vi "Bootstrapping.vi"() -> ()   [LabVIEW 2012]
panel:
  in  "bootstrap script":string="-- This is an example bootstrap script with the optional onfiguration\n-- actions and settings commented out.\n\n-- Substitution of \"\\\" and \"/\" in path strings with the platform path seperator\n-- is enabled by default. Uncomment the line below to disable this behaviour.\n--lv.substitute_separators(false)\n\n-- To globally tune auto-yielding, uncomment the line below and tweak\n-- the timing parameters.\n--lv.setyieldingdefaults(2,0)\n\n-- Specify various configuration settings. When a setting is commented out\n-- or omitted, its current/default value will be used. When the bootstrap\n-- script completes, any changes made to these settings will be reverted.\n-- These settings map to globals \"glb_LuaVIEW Configuration Globals.vi\"\n-- and \"glb_Library Configuration Globals.vi\". See the description of the\n-- variables contained therein for detailed documentation.\nconfigure({\n--[\"bootmode\"]=\"test\"\n--[\"resource base path\"]=lv.app_dir(),\n--[\"time format\"]=\"%Y/%m/%d %H:%M:%S\",\n--[\"persistence path\"]=\"great app\",\n--[\"auto-init registry\"]=true,\n--[\"unload functions ASAP\"]=(app_kind()==\"Run Time System\"),\n--[\"script search directories\"]={\"imports/libraries\",\"imports/configs\"},\n--[\"custom info\"]=\"My great application. (C) GreatWare Inc.\",\n--[\"export timeout\"]=1000,\n--[\"incite timeout\"]=1000,\n--[\"mandatory import script\"]=[[]],\n--[\"task error logger\"]=\"\",\n})\n\n-- Register a selection of public LuaVIEW functions.\nif app_kind()~=\"Run Time System\" then\n    register.public_dir(\"luaview/functions\")\nend\n\n-- Now we can start a script that can assume a proper configuration\n-- and use the public functions that were registered.\n-- Note that a script file can be used instead of an in-line script.\ndo_script(\"startup\",[[\nprint(\"Hello world!\")\nwait(2000)\nprint(\"Goodbye cruel world...\")\n]])\n"
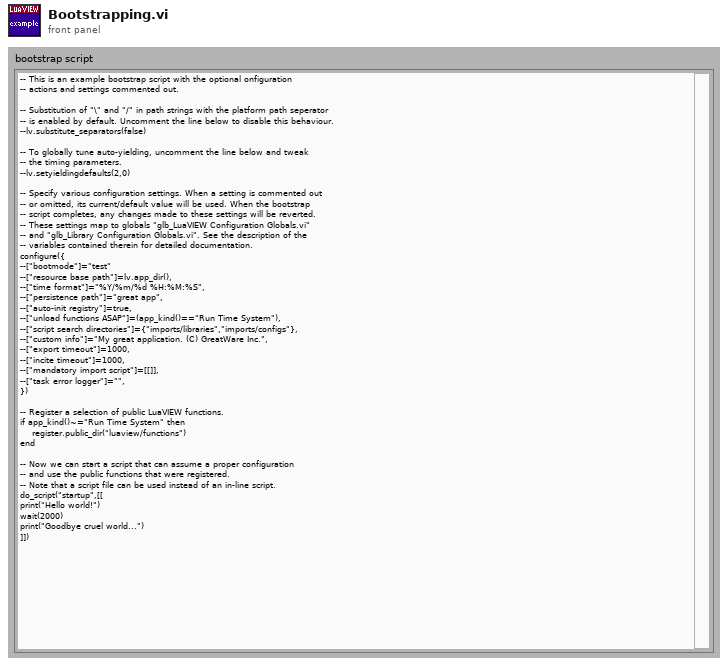
[diagram p1: front panel]
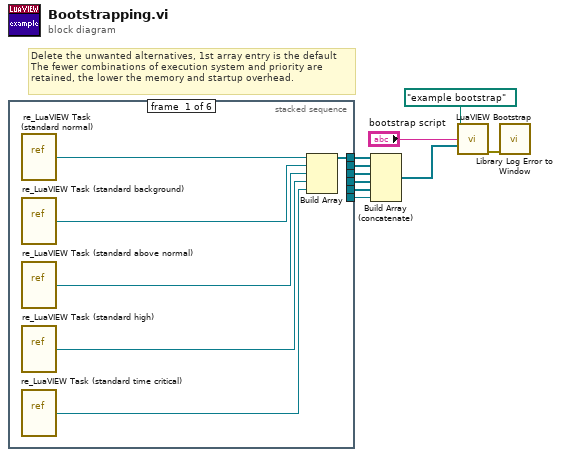
[diagram p0: block diagram]
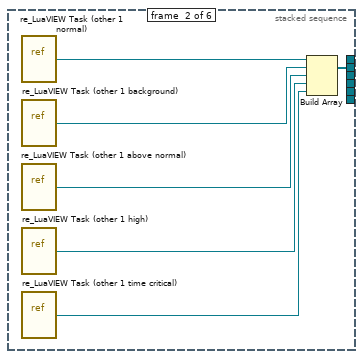
[diagram p2: hidden frame]
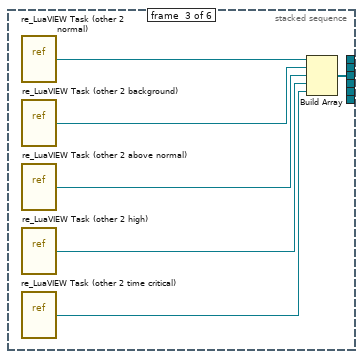
[diagram p3: hidden frame]
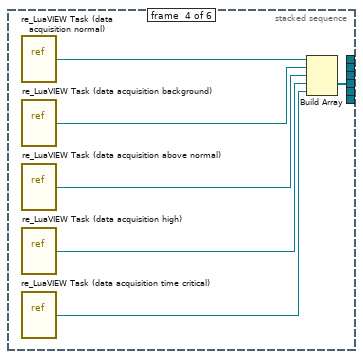
[diagram p4: hidden frame]
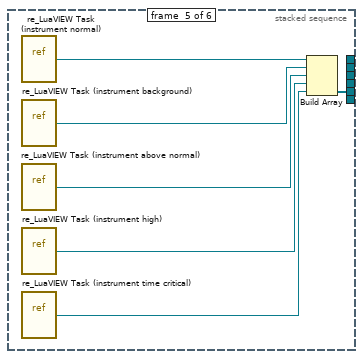
[diagram p5: hidden frame]
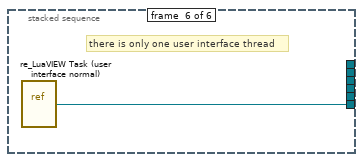
[diagram p6: hidden frame]
diagram:
  # "Delete the unwanted alternatives, 1st array entry is the default\nThe fewer combinations of execution system and priority are\nretained, the lower the memory and startup overhead."
  n1 = stacked-sequence {
    tunnel: [w11 _ _ _ _ _] -> w7
    tunnel: [_ w17 _ _ _ _] -> w6
    tunnel: [_ _ w23 _ _ _] -> w5
    tunnel: [_ _ _ w29 _ _] -> w4
    tunnel: [_ _ _ _ w35 _] -> w3
    tunnel: [_ _ _ _ _ w41] -> w2
    frame #0 {
      n2 = vi-ref "re_LuaVIEW Task (standard normal).vi"() -> ("vi reference"=w16:refnum<vi>)
      n3 = vi-ref "re_LuaVIEW Task (standard background).vi"() -> ("vi reference"=w15:refnum<vi>)
      n4 = vi-ref "re_LuaVIEW Task (standard above normal).vi"() -> ("vi reference"=w14:refnum<vi>)
      n5 = vi-ref "re_LuaVIEW Task (standard high).vi"() -> ("vi reference"=w13:refnum<vi>)
      n6 = vi-ref "re_LuaVIEW Task (standard time critical).vi"() -> ("vi reference"=w12:refnum<vi>)
      n7 = Build Array(w16, w15, w14, w13, w12) -> (w11:refnum<vi>[])
    }
    frame #1 {
      n8 = vi-ref "re_LuaVIEW Task (other 1 normal).vi"() -> ("vi reference"=w22:refnum<vi>)
      n9 = vi-ref "re_LuaVIEW Task (other 1 background).vi"() -> ("vi reference"=w21:refnum<vi>)
      n10 = vi-ref "re_LuaVIEW Task (other 1 above normal).vi"() -> ("vi reference"=w20:refnum<vi>)
      n11 = vi-ref "re_LuaVIEW Task (other 1 high).vi"() -> ("vi reference"=w19:refnum<vi>)
      n12 = vi-ref "re_LuaVIEW Task (other 1 time critical).vi"() -> ("vi reference"=w18:refnum<vi>)
      n13 = Build Array(w22, w21, w20, w19, w18) -> (w17:refnum<vi>[])
    }
    frame #2 {
      n14 = vi-ref "re_LuaVIEW Task (other 2 normal).vi"() -> ("vi reference"=w28:refnum<vi>)
      n15 = vi-ref "re_LuaVIEW Task (other 2 background).vi"() -> ("vi reference"=w27:refnum<vi>)
      n16 = vi-ref "re_LuaVIEW Task (other 2 above normal).vi"() -> ("vi reference"=w26:refnum<vi>)
      n17 = vi-ref "re_LuaVIEW Task (other 2 high).vi"() -> ("vi reference"=w25:refnum<vi>)
      n18 = vi-ref "re_LuaVIEW Task (other 2 time critical).vi"() -> ("vi reference"=w24:refnum<vi>)
      n19 = Build Array(w28, w27, w26, w25, w24) -> (w23:refnum<vi>[])
    }
    frame #3 {
      n20 = vi-ref "re_LuaVIEW Task (data acquisition normal).vi"() -> ("vi reference"=w34:refnum<vi>)
      n21 = vi-ref "re_LuaVIEW Task (data acquisition background).vi"() -> ("vi reference"=w33:refnum<vi>)
      n22 = vi-ref "re_LuaVIEW Task (data acquisition above normal).vi"() -> ("vi reference"=w32:refnum<vi>)
      n23 = vi-ref "re_LuaVIEW Task (data acquisition high).vi"() -> ("vi reference"=w31:refnum<vi>)
      n24 = vi-ref "re_LuaVIEW Task (data acquisition time critical).vi"() -> ("vi reference"=w30:refnum<vi>)
      n25 = Build Array(w34, w33, w32, w31, w30) -> (w29:refnum<vi>[])
    }
    frame #4 {
      n26 = vi-ref "re_LuaVIEW Task (instrument normal).vi"() -> ("vi reference"=w40:refnum<vi>)
      n27 = vi-ref "re_LuaVIEW Task (instrument background).vi"() -> ("vi reference"=w39:refnum<vi>)
      n28 = vi-ref "re_LuaVIEW Task (instrument above normal).vi"() -> ("vi reference"=w38:refnum<vi>)
      n29 = vi-ref "re_LuaVIEW Task (instrument high).vi"() -> ("vi reference"=w37:refnum<vi>)
      n30 = vi-ref "re_LuaVIEW Task (instrument time critical).vi"() -> ("vi reference"=w36:refnum<vi>)
      n31 = Build Array(w40, w39, w38, w37, w36) -> (w35:refnum<vi>[])
    }
    frame #5 {
      # "there is only one user interface thread"
      n32 = vi-ref "re_LuaVIEW Task (user interface normal).vi"() -> ("vi reference"=w41:refnum<vi>)
    }
  }
  n33 = Build Array (concatenate)(w7, w6, w5, w4, w3, w2) -> (w1:refnum<vi>[])
  n34 = call "LuaVIEW Bootstrap.vi"("script file or name (no name)"=path "example bootstrap", "script string (\"\" == load from file)"="bootstrap script", "task alternatives (default)"=w1) -> ("error out"=w9:errorcluster)  [unwired: 12 in]
  n35 = call "Library Log Error to Window.vi"("error in (no error)"=w9) -> ()  [unwired: 13 in, 2 out]
